vi "Test Config File.vi"() -> ()   [LabVIEW 2020]
panel:
  out "Variant array":variant[](array[variant])
  in  "Coil":enum16{"HTS", "LTS"}(ring)=enum."LTS"
  in  "Config data":variant[](array[variant])
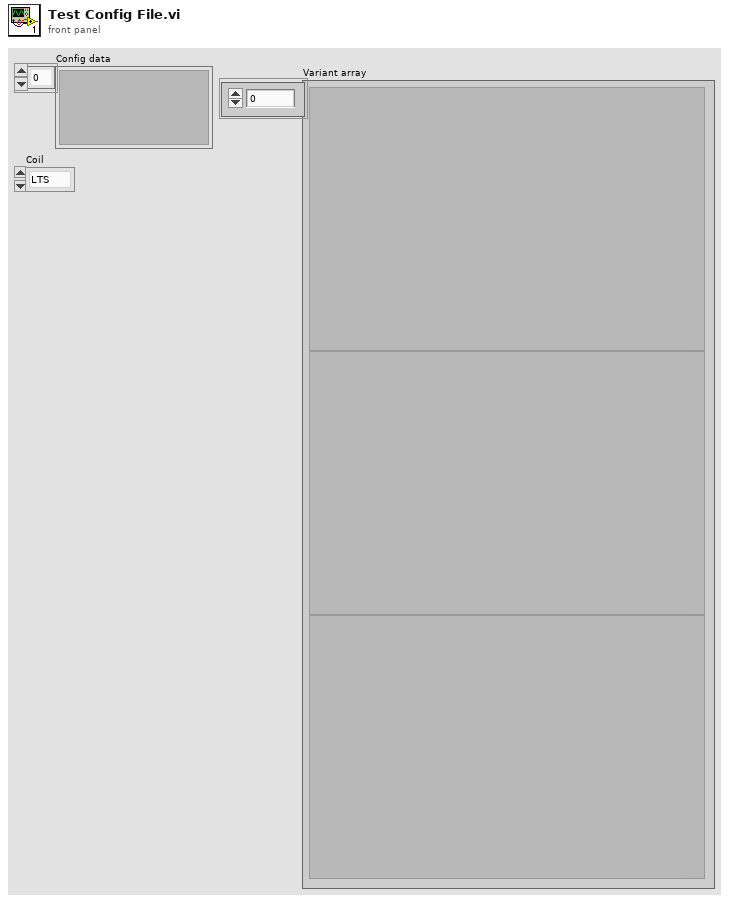
[diagram p1: front panel]
types:
  T1 = typedef "NI_LVConfig.lvlib/Config Data RefNum.ctl" = refnum<k1>
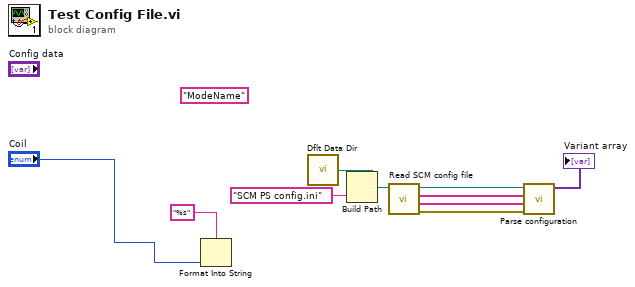
[diagram p0: block diagram]
diagram:
  (unwired) "ModeName"
  n1 = Format Into String(format string="%s", "Coil") -> ()  [unwired: 2 in, 2 out]
  n2 = call <vilib>:"Dflt Data Dir.vi"() -> ("App:Default Data Directory"=w4:path)
  n3 = Build Path(base path=w4, name or relative path="SCM PS config.ini") -> (appended path=w2:path)
  n4 = call "Read SCM config file.vi"("appended path"=w2) -> ("error out"=w5:errorcluster, "Array"=w6:string[], "Array 2"=w7:string[], "Refnum out"=w8:T1)  [unwired: 7 in]
  n5 = call "Parse configuration.vi"("error in (no error)"=w5, "Mode Name for Variant"=w6, "Config File Sections"=w7, "Refnum in"=w8) -> ("Variant array"=→"Variant array":variant[])  [unwired: 6 in, 1 out]
